vi "WELCOME SCREEN.MAIN.vi"() -> ()   [LabVIEW 2026]
panel:
  in  "WELCOME":bool
  out "2D Picture":picture
  in  "Combo Box":string(combo)="WELCOME.PNG"
  in  "Enum":enum16{"PNG", "JPEG"}(ring)
  in  "stop":bool
  out "error constant 2":errorcluster
  in  "error constant":errorcluster
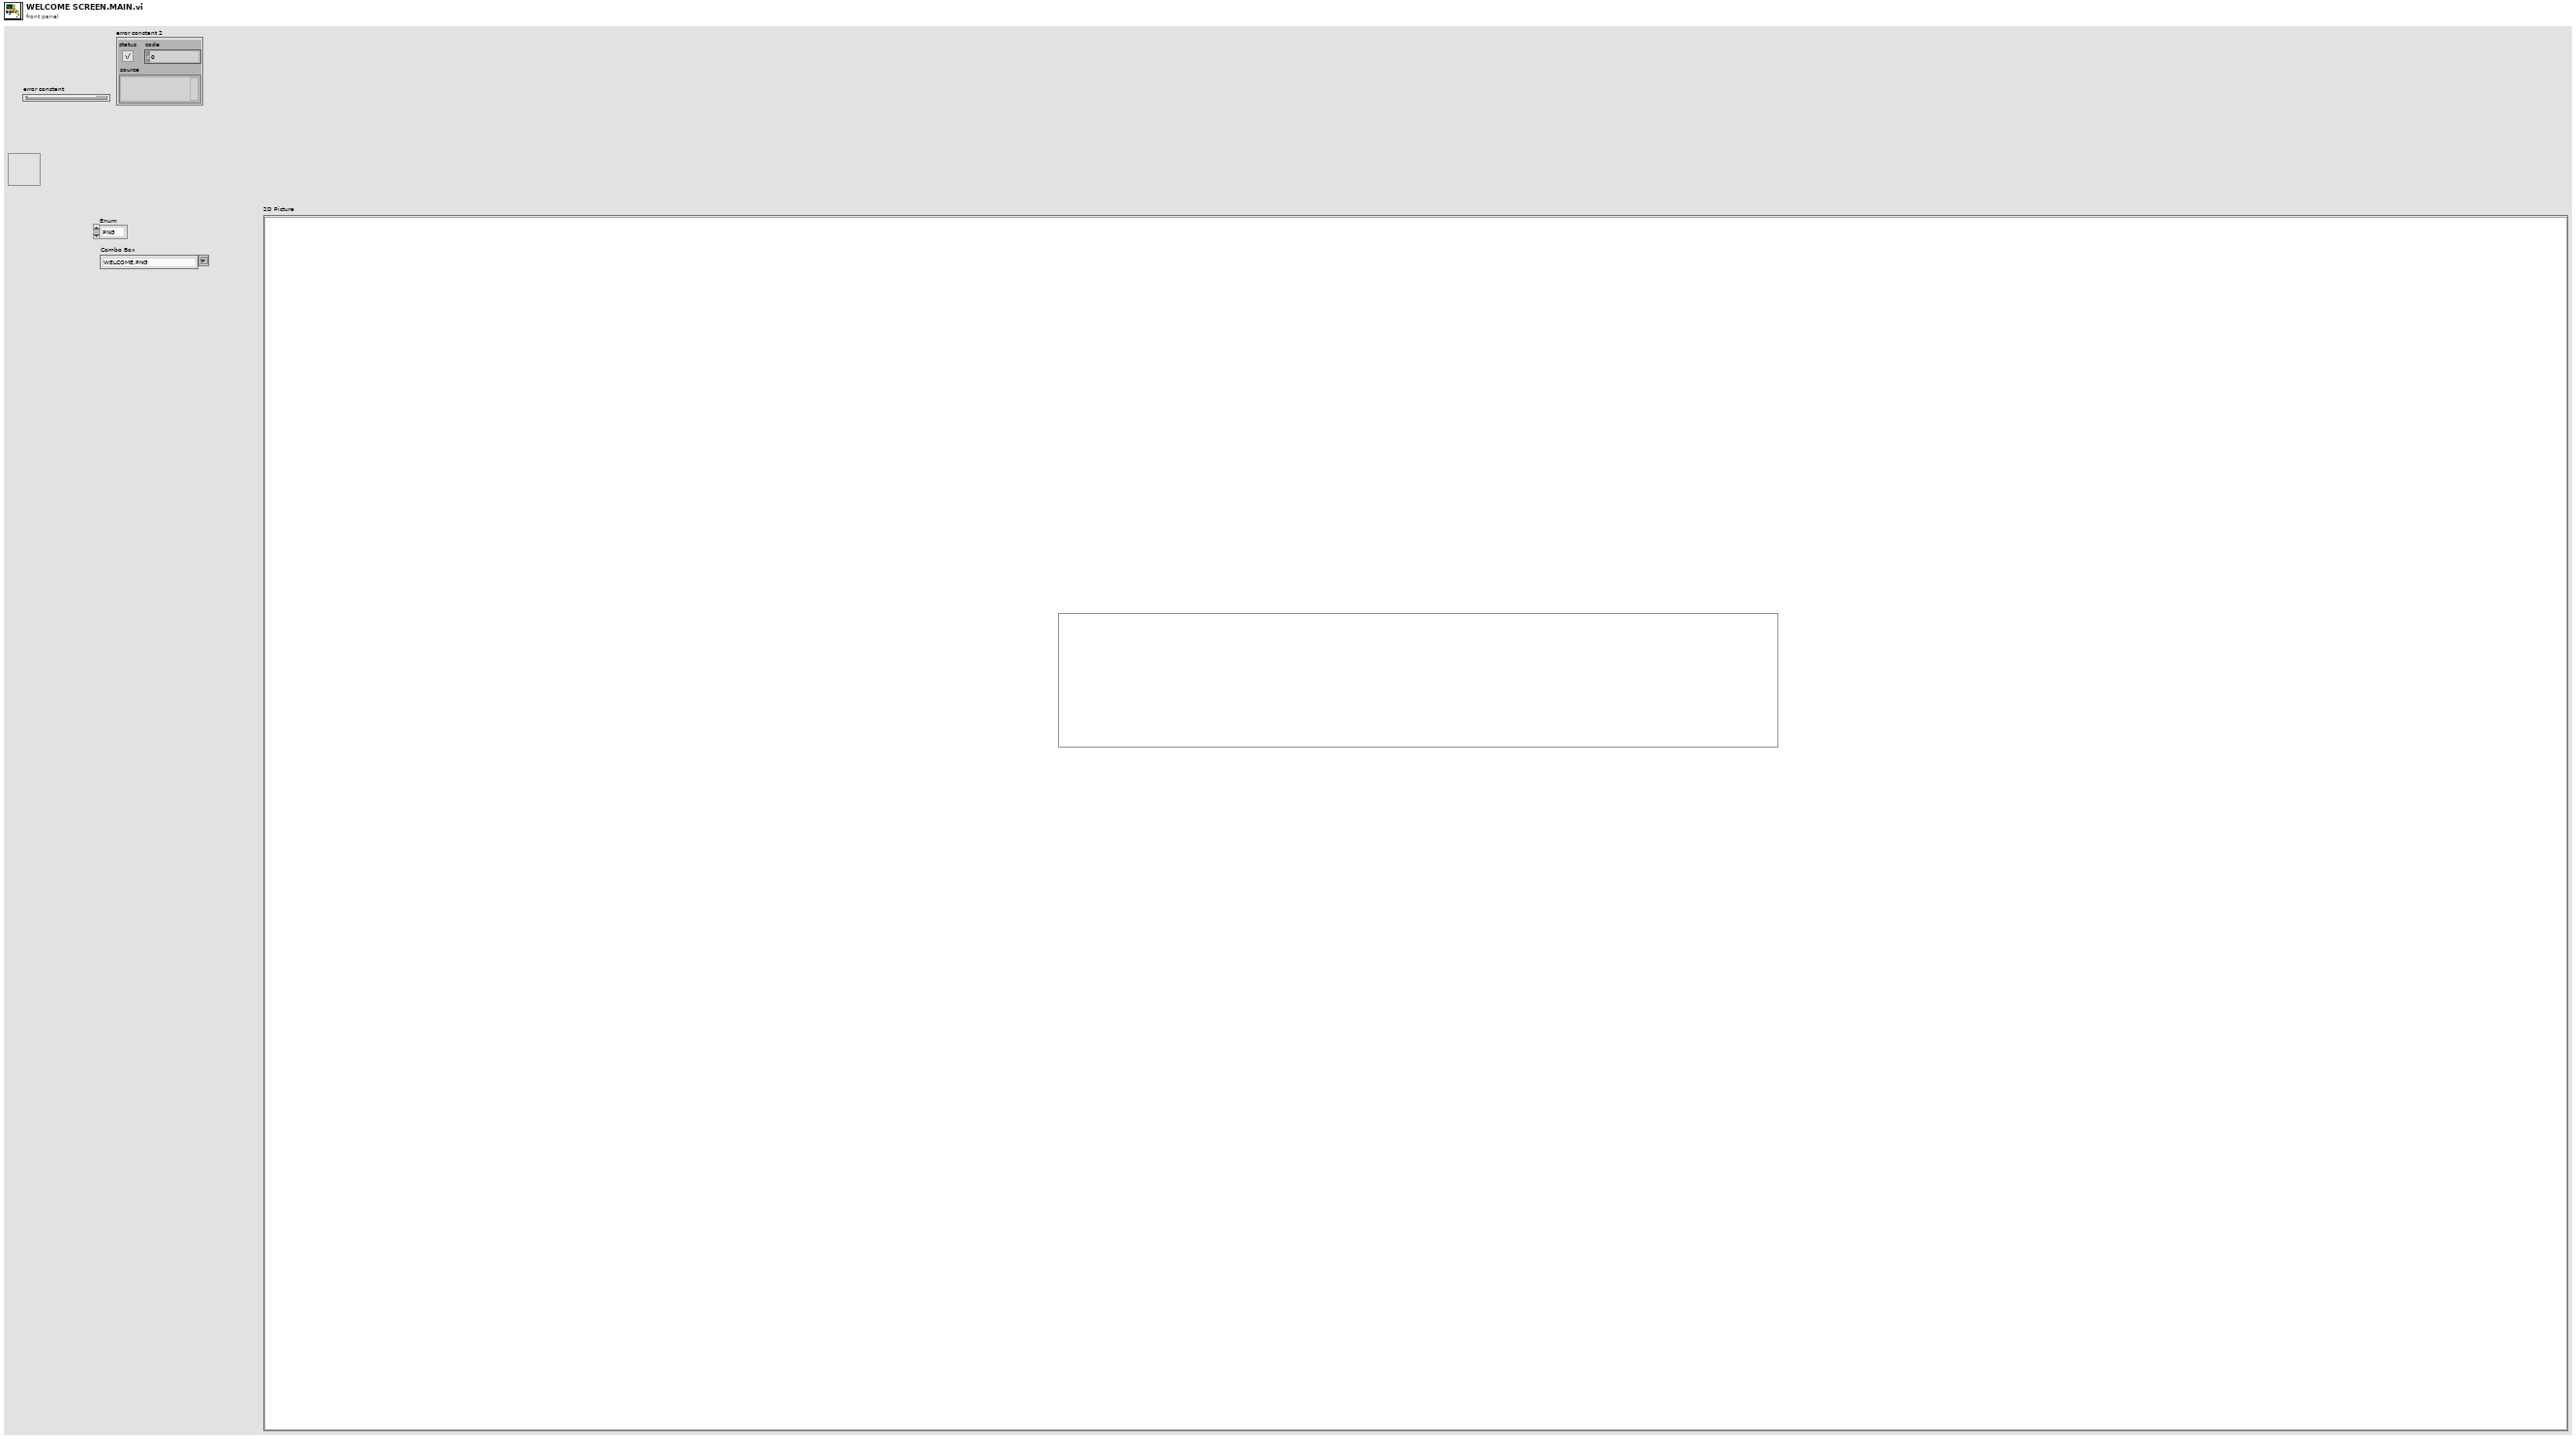
[diagram p1: front panel]
types:
  T1 = typedef "imagedata.ctl" = cluster{"image type":i32, "image depth":i32, "image":u8[], "mask":u8[], "colors":u32[], "Rectangle":cluster{"left":i16, "top":i16, "right":i16, "bottom":i16}}
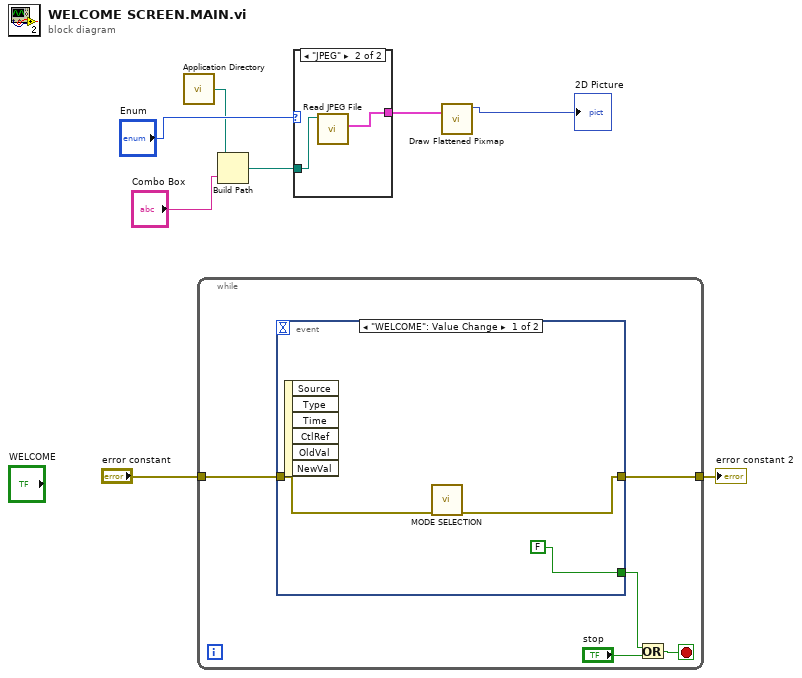
[diagram p0: block diagram]
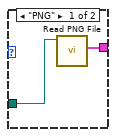
[diagram p2: hidden frame]
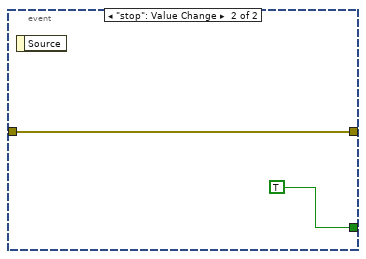
[diagram p3: hidden frame]
diagram:
  n1 = call <vilib>:"Application Directory.vi"() -> ("Application Directory"=w4:path)
  n2 = while {
    tunnel: "error constant" -> [w11]
    tunnel: [w10] -> w7
    stop <- w9 stop-if-true
    n3 = event shown="[0] \"WELCOME\": Value Change" {
      selector: _ -> [_ _]
      dyn-events: _ -> [_ _]
      timeout: _ -> [_ _]
      tunnel: [FALSE TRUE] -> w12
      tunnel: w11 -> [w15 w17]
      tunnel: [w14 w17] -> w10
      event "WELCOME": Value Change {
        n4 = event-data() -> ()  [unwired: 1 in, 6 out]
        n5 = call "MODE SELECTION.vi"("error constant"=w15) -> ("error constant 2"=w14:errorcluster)  [unwired: 10 in]
      }
      event "stop": Value Change {
        n6 = event-data() -> ()  [unwired: 1 in, 1 out]
      }
    }
    n7 = Or(x=w12, y="stop") -> (x .or. y?=w9:bool)
  }
  "error constant 2" <- w7
  n8 = Build Path(base path=w4, name or relative path="Combo Box") -> (appended path=w5:path)
  n9 = case shown="\"JPEG\"" "Enum" {
    tunnel: w5 -> [w20 w21]
    tunnel: [w19 w22] -> w2
    frame "PNG" {
      n10 = call <vilib>:"Read PNG File.vi"("path to PNG file"=w20) -> ("image data"=w19:T1)  [unwired: 8 in, 2 out]
    }
    frame "JPEG" {
      n11 = call <vilib>:"Read JPEG File.vi"("path to JPEG file"=w21) -> ("image data"=w22:T1)  [unwired: 8 in, 2 out]
    }
  }
  n12 = call <vilib>:"Draw Flattened Pixmap.vi"("image data"=w2) -> ("new picture"=→"2D Picture":picture)  [unwired: 8 in]
